vi "Ballard - 1553 - Main Page.vi"(8 "error in (no error)":errorcluster, 11 "Node Ptr":T2 format="%.0x") -> (0 "error out":errorcluster)   [LabVIEW 2017, in "Ballard 1553 System Explorer.lvlib"]
uses:
  Ballard 1553 System Explorer.lvlib
  <vilib>/NI Veristand/Custom Device API/Custom Device Item Ref.ctl
  Shared/Controls and Global/Initialization Method.ctl
  Shared/Controls and Global/Global.vi
  <vilib>/NI Veristand/Custom Device API/Get Item Property (U16).vi
  <vilib>/NI Veristand/Custom Device API/Get Item Property (I32).vi
  <vilib>/NI Veristand/Custom Device API/Get Item Property (Path).vi
  <vilib>/NI Veristand/Custom Device API/Get Item Property (String).vi
  <vilib>/NI Veristand/Custom Device API/Set Item Property (I32).vi
  <vilib>/NI Veristand/Custom Device API/Set Item Property (U16).vi
  <vilib>/NI VeriStand/Custom Device API/Custom Device API.lvlib
  Shared/Ballard 1553 Shared.lvlib
panel:
  in  "PXI Slot Number":i32=1 min=1 max=18 step=1
  in  "Initialization Method":T1
  out "Parameters Configuration Warning text":string="WARNING: The Parameters Configuration File has changed since import. If you attempt to run this system definition an error may occur. Consider refreshing the database import."
  out "Parameters Configuration File":path
  in  "Core Number":i32
  in  "Card Number":i32 min=0 max=18 step=1
  out "Version":string
  out "HW Configuration Warning text":string="WARNING: The database has changed since import. If you attempt to run this system definition an error may occur. Consider refreshing the database import."
  out "Warn Icon":bool
  out "Hardware Configuration File":path
  in  "Header":cluster{"Section Name":string}={"Section Name"="Ballard - MIL-STD-1553 - Custom Device"}
  in  "Description":string
  in  "Name":string
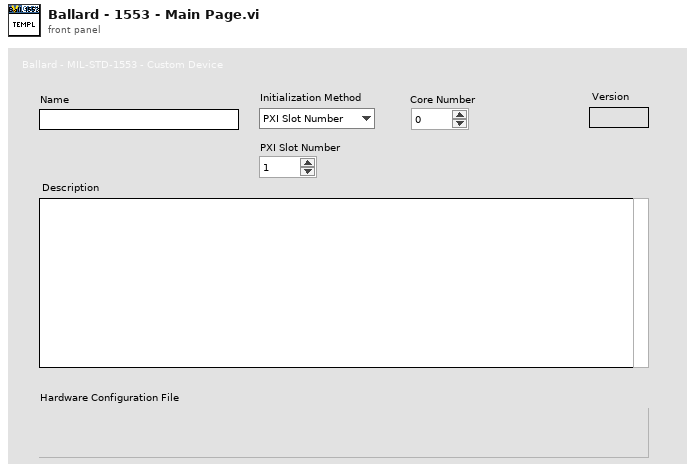
[diagram p1: front panel]
types:
  T1 = typedef "Ballard 1553 Shared.lvlib/Initialization Method.ctl" = enum16{"PXI Slot Number", "Card Number"}
  T2 = typedef "Custom Device API.lvlib/Custom Device Item Ref.ctl" = u64
  T3 = typedef "Custom Device API.lvlib/Custom Device Item Info.ctl" = cluster{"Name":string, "Is Channel":bool, "GUID":string, "Is Waveform":bool}
  T4 = typedef "Custom Device API.lvlib/Custom Device Commands.ctl" = enum16{"Default", "Item renamed", "Shutdown", "Dynamic button pressed"}
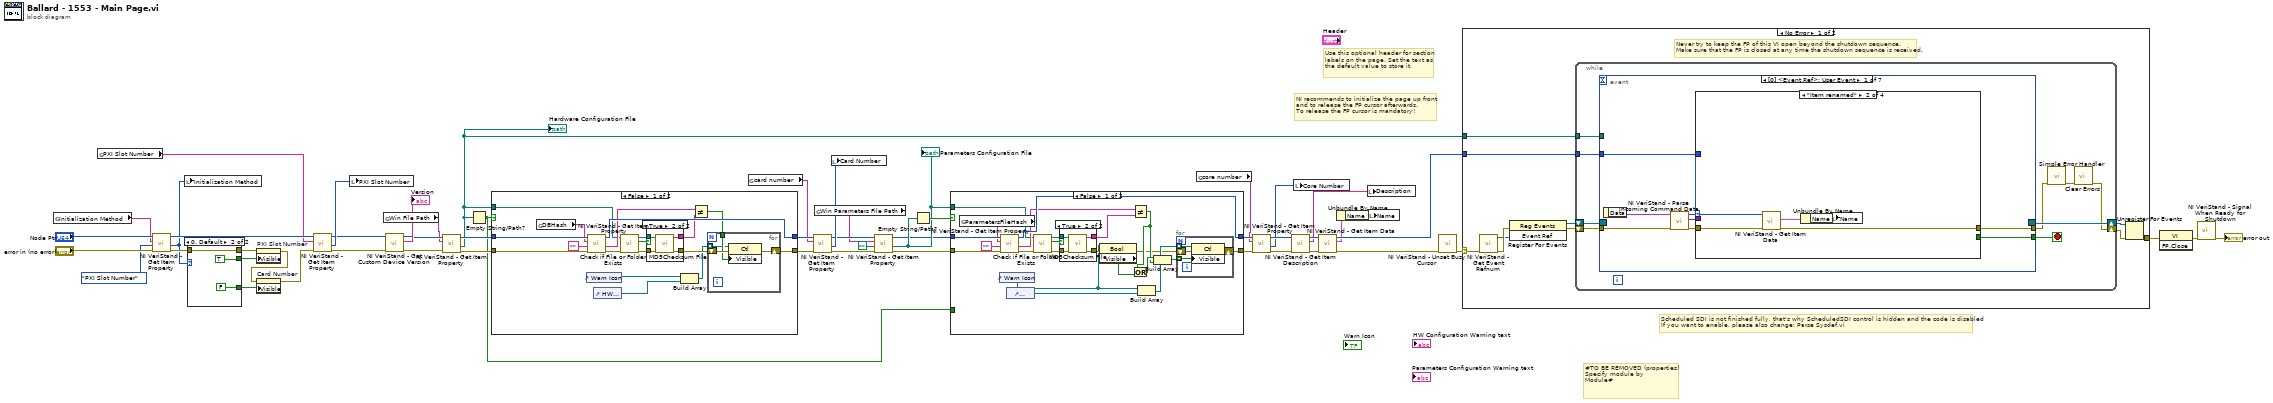
[diagram p0: block diagram]
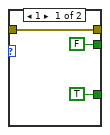
[diagram p2: hidden frame]
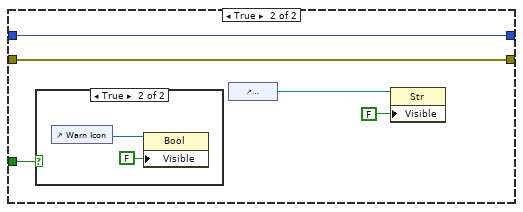
[diagram p4: hidden frame]
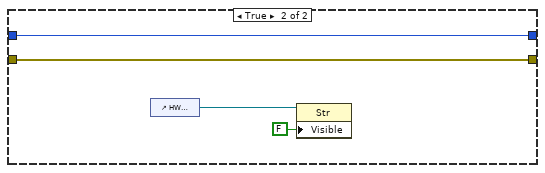
[diagram p7: hidden frame]
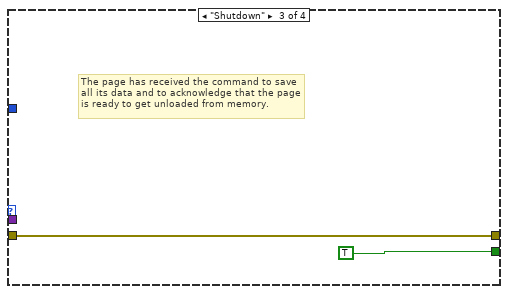
[diagram p9: hidden frame]
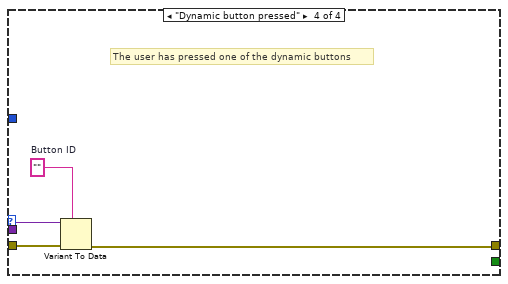
[diagram p10: hidden frame]
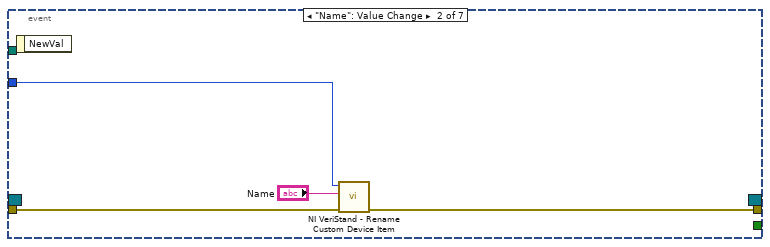
[diagram p11: hidden frame]
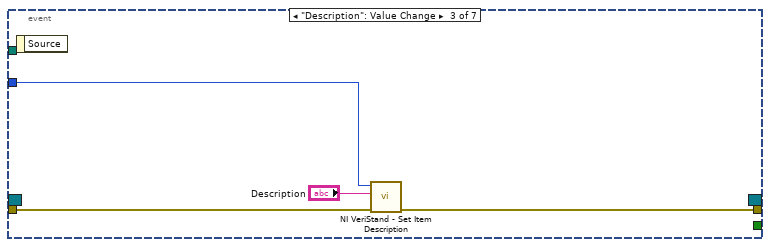
[diagram p12: hidden frame]
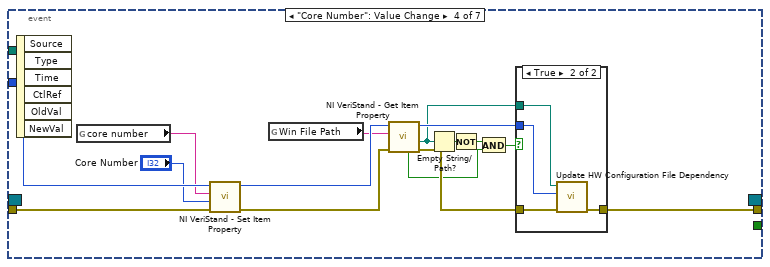
[diagram p13: hidden frame]
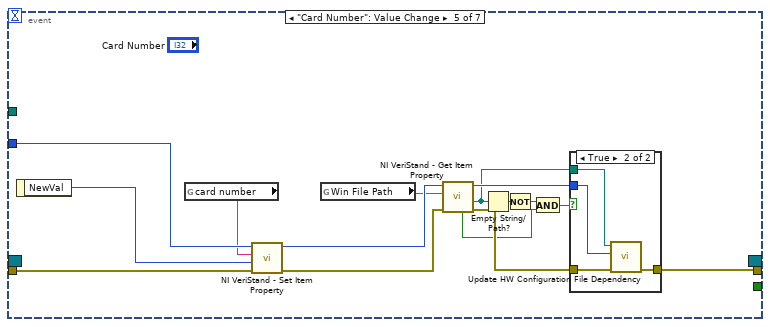
[diagram p15: hidden frame]
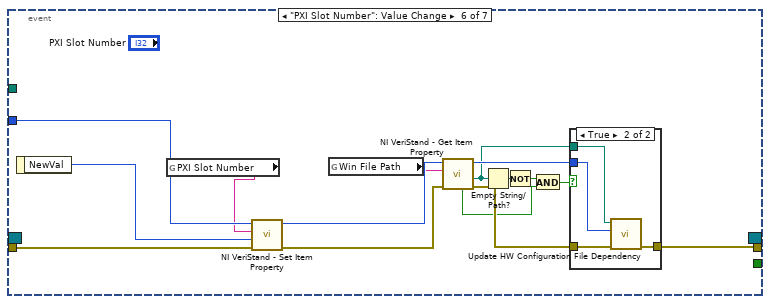
[diagram p17: hidden frame]
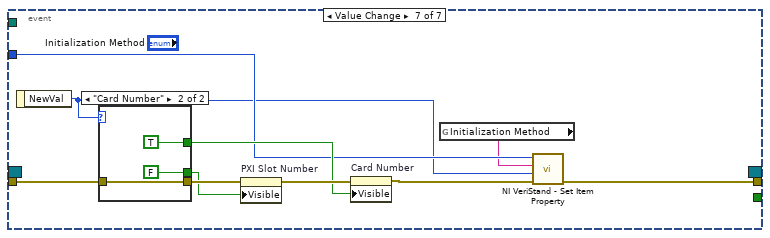
[diagram p19: hidden frame]
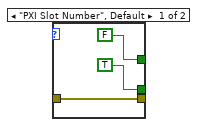
[diagram p20: hidden frame]
diagram:
  # "#TO BE REMOVED (properties)\nSpecify module by\nModule#"
  # "Scheduled SDI is not finished fully, that's why ScheduledSDI control is hidden and the code is disabled\nIf you want to enable, please also change: Parse Sysdef.vi"
  # "Use this optional header for section labels on the page. Set the text as the default value to store it."
  # "NI recommends to initialize the page up front\nand to release the FP cursor afterwards.\nTo release the FP cursor is mandatory!"
  n1 = global read "Global.vi" "Initialization Method"() -> (w5:string)
  n2 = global read "Global.vi" "PXI Slot Number"() -> (w6:string)
  n3 = call-poly <vilib>:"NI VeriStand - Get Item Property.vi"("error in (no error)"="error in (no error)", "Default Value"=Initialization_Method."PXI Slot Number" ("Initialization Method"), "Property Name"=w5, "Item Ref in"="Node Ptr") -> ("error out"=w13:errorcluster, "Value"=w12:u16, "Item Ref out"=w20:T2)  [unwired: 4 in, 1 out]
  n4 = local write "Initialization Method"(w12) -> ()
  n5 = case shown="0, Default" w12 {
    tunnel: w13 -> [w56 w59]
    tunnel: [FALSE TRUE] -> w11
    tunnel: [w56 w59] -> w10
    tunnel: [TRUE FALSE] -> w7
    frame 1 {
    }
    frame 0, Default {
    }
  }
  n6 = property on="PXI Slot Number" class="DigNum (strict)"(error in=w10, "Visible"=w11) -> (error out=w9:errorcluster)  [unwired: 1 in, 1 out]
  n7 = property on="Card Number" class="DigNum (strict)"(error in=w9, "Visible"=w7) -> (error out=w8:errorcluster)  [unwired: 1 in, 1 out]
  n8 = call-poly <vilib>:"NI VeriStand - Get Item Property.vi"("error in (no error)"=w8, "Property Name"=w6, "Item Ref in"=w20) -> ("error out"=w14:errorcluster, "Value"=w16:i32, "Item Ref out"=w15:T2)  [unwired: 5 in, 1 out]
  n9 = local write "PXI Slot Number"(w16) -> ()
  n10 = global read "Global.vi" "Win File Path"() -> (w4:string)
  n11 = call <vilib>:"NI VeriStand - Get Custom Device Version.vi"("error in (no error)"=w14, "Device Ref in"=w15) -> ("error out"=w35:errorcluster, "Value"=→"Version":string, "Device Ref out"=w36:T2)  [unwired: 7 in]
  n12 = call-poly <vilib>:"NI VeriStand - Get Item Property.vi"("error in (no error)"=w35, "Property Name"=w4, "Item Ref in"=w36) -> ("error out"=w42:errorcluster, "Value"=w38:path, "Item Ref out"=w39:T2)  [unwired: 5 in, 1 out]
  "Hardware Configuration File" <- w38
  n13 = Empty String/Path?(string/path=w38) -> (empty?=w21:bool)
  n14 = case shown="False" w21 {
    tunnel: w42 -> [w75 w90]
    tunnel: [w66 w90] -> w41
    tunnel: [w74 w89] -> w40
    tunnel: w39 -> [w76 w89]
    tunnel: w38 -> [w62 _]
    frame False {
      n15 = global read "Global.vi" "DBHash"() -> (w60:string)
      n16 = control-ref of="Warn Icon"() -> (w68:refnum<vi>)
      n17 = call-poly <vilib>:"NI VeriStand - Get Item Property.vi"("error in (no error)"=w75, "Default Value"="", "Property Name"=w60, "Item Ref in"=w76) -> ("error out"=w63:errorcluster, "Value"=w72:string, "Item Ref out"=w74:T2)  [unwired: 4 in, 1 out]
      n18 = control-ref of="HW Configuration Warning text"() -> (w69:refnum<vi>)
      n19 = call <vilib>:"Check if File or Folder Exists.vi"("error in (no error)"=w63, "path"=w62) -> ("error out"=w65:errorcluster, "file or folder exists?"=w61:bool, "dup path"=w64:path)  [unwired: 7 in]
      n20 = case shown="True" w61 {
        tunnel: [_ w82] -> w73
        tunnel: [w78 w81] -> w71
        tunnel: w65 -> [w78 w80]
        tunnel: w64 -> [_ w79]
        frame False {
        }
        frame True {
          n21 = call <vilib>:"MD5Checksum File.vi"("error in (no error)"=w80, "Path"=w79) -> ("error out"=w81:errorcluster, "MD5 message-digest"=w82:string)  [unwired: 8 in]
        }
      }
      n22 = Build Array(w68, w69) -> (w67:refnum<vi>[])
      n23 = Not Equal?(x=w72, y=w73) -> (x != y?=w70:bool)
      n24 = for {
        shift-right: [w85] -> w66
        shift-left: w71 -> [w86]
        tunnel: w70 -> [w84]
        tunnel: w67 -> [w83] mode=indexing
        n25 = property class="Ctl"(reference=w83, error in=w86, "Visible"=w84) -> (error out=w85:errorcluster)  [unwired: 1 out]
      }
    }
    frame True {
      n26 = control-ref of="HW Configuration Warning text"() -> (w88:refnum<vi>)
      n27 = property class="Str"(reference=w88, "Visible"=FALSE) -> ()  [unwired: 1 in, 2 out]
    }
  }
  n28 = global read "Global.vi" "card number"() -> (w3:string)
  n29 = call-poly <vilib>:"NI VeriStand - Get Item Property.vi"("error in (no error)"=w41, "Property Name"=w3, "Item Ref in"=w40) -> ("error out"=w29:errorcluster, "Value"=w31:i32, "Item Ref out"=w30:T2)  [unwired: 5 in, 1 out]
  n30 = global read "Global.vi" "Win Parameters File Path"() -> (w2:string)
  n31 = local write "Card Number"(w31) -> ()
  n32 = call-poly <vilib>:"NI VeriStand - Get Item Property.vi"("error in (no error)"=w29, "Default Value"=path "", "Property Name"=w2, "Item Ref in"=w30) -> ("error out"=w24:errorcluster, "Value"=w27:path, "Item Ref out"=w26:T2)  [unwired: 4 in, 1 out]
  "Parameters Configuration File" <- w27
  n33 = Empty String/Path?(string/path=w27) -> (empty?=w28:bool)
  n34 = case shown="False" w28 {
    tunnel: [w107 w125] -> w23
    tunnel: [w110 w126] -> w25
    tunnel: w26 -> [w111 w126]
    tunnel: w27 -> [w103 _]
    tunnel: w24 -> [w92 w125]
    tunnel: w21 -> [_ w122]
    frame False {
      n35 = global read "Global.vi" "ParametersFileHash"() -> (w91:string)
      n36 = control-ref of="Warn Icon"() -> (w93:refnum<vi>)
      n37 = call-poly <vilib>:"NI VeriStand - Get Item Property.vi"("error in (no error)"=w92, "Default Value"="", "Property Name"=w91, "Item Ref in"=w111) -> ("error out"=w104:errorcluster, "Value"=w108:string, "Item Ref out"=w110:T2)  [unwired: 4 in, 1 out]
      n38 = control-ref of="Parameters Configuration Warning text"() -> (w101:refnum<vi>)
      n39 = call <vilib>:"Check if File or Folder Exists.vi"("error in (no error)"=w104, "path"=w103) -> ("error out"=w106:errorcluster, "file or folder exists?"=w102:bool, "dup path"=w105:path)  [unwired: 7 in]
      n40 = case shown="True" w102 {
        tunnel: [_ w121] -> w109
        tunnel: [w117 w120] -> w98
        tunnel: w106 -> [w117 w119]
        tunnel: w105 -> [_ w118]
        frame False {
        }
        frame True {
          n41 = call <vilib>:"MD5Checksum File.vi"("error in (no error)"=w119, "Path"=w118) -> ("error out"=w120:errorcluster, "MD5 message-digest"=w121:string)  [unwired: 8 in]
        }
      }
      n42 = property class="Bool"(reference=w93, error in=w98) -> (error out=w94:errorcluster, "Visible"=w96:bool)  [unwired: 1 out]
      n43 = Not Equal?(x=w108, y=w109) -> (x != y?=w95:bool)
      n44 = Or(x=w95, y=w96) -> (x .or. y?=w97:bool)
      n45 = Build Array(w93, w101) -> (w100:refnum<vi>[])
      n46 = Build Array(w97, w95) -> (w99:bool[])
      n47 = for {
        tunnel: w99 -> [w114] mode=indexing
        shift-right: [w115] -> w107
        shift-left: w94 -> [w116]
        tunnel: w100 -> [w113] mode=indexing
        n48 = property class="Ctl"(reference=w113, error in=w116, "Visible"=w114) -> (error out=w115:errorcluster)  [unwired: 1 out]
      }
    }
    frame True {
      n49 = case shown="True" w122 {
        frame False {
        }
        frame True {
          n50 = control-ref of="Warn Icon"() -> (w128:refnum<vi>)
          n51 = property class="Bool"(reference=w128, "Visible"=FALSE) -> ()  [unwired: 1 in, 2 out]
        }
      }
      n52 = control-ref of="Parameters Configuration Warning text"() -> (w124:refnum<vi>)
      n53 = property class="Str"(reference=w124, "Visible"=FALSE) -> ()  [unwired: 1 in, 2 out]
    }
  }
  n54 = global read "Global.vi" "core number"() -> (w1:string)
  n55 = call-poly <vilib>:"NI VeriStand - Get Item Property.vi"("error in (no error)"=w23, "Property Name"=w1, "Item Ref in"=w25) -> ("error out"=w34:errorcluster, "Value"=w32:i32, "Item Ref out"=w33:T2)  [unwired: 5 in, 1 out]
  n56 = call <vilib>:"NI VeriStand - Get Item Description.vi"("error in (no error)"=w34, "Item Ref in"=w33) -> ("error out"=w45:errorcluster, "Description"=w46:string, "Item Ref out"=w47:T2)  [unwired: 7 out]
  n57 = local write "Core Number"(w32) -> ()
  n58 = call <vilib>:"NI VeriStand - Get Item Data.vi"("error in (no error)"=w45, "Item Ref in"=w47) -> ("error out"=w50:errorcluster, "Item Info"=w44:T3, "Item Ref out"=w48:T2)  [unwired: 7 out]
  n59 = Unbundle By Name(w44) -> ("Name"=w43:string)
  n60 = local write "Description"(w46) -> ()
  n61 = local write "Name"(w43) -> ()
  n62 = call <vilib>:"NI VeriStand - Unset Busy Cursor.vi"("error in (no error)"=w50) -> ("error out"=w49:errorcluster)  [unwired: 10 out]
  n63 = case shown="No Error" w49 {
    selector: w49 -> [w130 w254]
    tunnel: [w135 w252] -> w53
    tunnel: w48 -> [w131 _]
    tunnel: w38 -> [w129 _]
    frame No Error {
      # "Never try to keep the FP of this VI open beyond the shutdown sequence.\nMake sure that the FP is closed at any time the shutdown sequence is received."
      n64 = call <vilib>:"NI VeriStand - Get Event Refnum.vi"("error in (no error)"=w130) -> ("error out"=w138:errorcluster, "Event Ref"=w134:refnum<user-event>)  [unwired: 9 out]
      n65 = register-events(error in=w138, w134) -> (reference out=w132:refnum<event-registration>, error out=w133:errorcluster)  [unwired: 1 in]
      n66 = while {
        tunnel: w131 -> [w143]
        shift-right: [w140] -> w136
        shift-left: w133 -> [w146]
        shift-right: [w147] -> w137
        shift-left: w132 -> [w145]
        tunnel: w129 -> [w139]
        stop <- w144 stop-if-true
        n67 = event shown="[0] <Event Ref>: User Event" {
          selector: w145 -> [_ _ _ _ _ _ _]
          dyn-events: [_ _ _ _ _ _ _] -> w147
          timeout: _ -> [_ _ _ _ _ _ _]
          tunnel: w146 -> [w155 w171 w174 w190 w210 w230 w245]
          tunnel: [w151 _ _ _ _ _ _] -> w144
          tunnel: [w150 w170 w173 w179 w203 w223 w237] -> w142
          tunnel: w143 -> [w149 w169 w175 w189 w209 w229 w240]
          tunnel: w139 -> [_ _ _ _ _ _ _]
          event User Event {
            n68 = event-data() -> ("Data"=w154:string)  [unwired: 1 out]
            n69 = call <vilib>:"NI VeriStand - Parse Incoming Command Data.vi"("error in (no error)"=w155, "Incoming data"=w154) -> ("error out"=w153:errorcluster, "Outgoing data"=w148:variant, "Action"=w152:T4)  [unwired: 7 out]
            n70 = case shown="\"Item renamed\"" w152 {
              tunnel: w153 -> [w156 w161 w162 w167]
              tunnel: [_ _ TRUE _] -> w151
              tunnel: [w156 w158 w162 w164] -> w150
              tunnel: w149 -> [_ w160 _ _]
              tunnel: w148 -> [_ _ _ w166]
              frame "Default", Default {
              }
              frame "Item renamed" {
                n71 = call <vilib>:"NI VeriStand - Get Item Data.vi"("error in (no error)"=w161, "Item Ref in"=w160) -> ("error out"=w158:errorcluster, "Item Info"=w159:T3)  [unwired: 8 out]
                n72 = Unbundle By Name(w159) -> ("Name"=w157:string)
                n73 = local write "Name"(w157) -> ()
              }
              frame "Shutdown" {
                # "The page has received the command to save all its data and to acknowledge that the page is ready to get unloaded from memory."
              }
              frame "Dynamic button pressed" {
                w165 = ""  # Button ID
                # "The user has pressed one of the dynamic buttons"
                n74 = Variant To Data(error in=w167, type=w165, Variant=w166) -> (error out=w164:errorcluster)  [unwired: 1 out]
              }
            }
          }
          event "Name": Value Change {
            n75 = event-data() -> ()  [unwired: 2 out]
            n76 = call <vilib>:"NI VeriStand - Rename Custom Device Item.vi"("error in (no error)"=w171, "New Name"="Name", "Item Ref in"=w169) -> ("error out"=w170:errorcluster)  [unwired: 1 in, 7 out]
          }
          event "Description": Value Change {
            n77 = event-data() -> ()  [unwired: 2 out]
            n78 = call <vilib>:"NI VeriStand - Set Item Description.vi"("error in (no error)"=w174, "Description"="Description", "Item Ref in"=w175) -> ("error out"=w173:errorcluster)  [unwired: 8 out]
          }
          event "Core Number": Value Change {
            n79 = event-data() -> ()  [unwired: 7 out]
            n80 = global read "Global.vi" "core number"() -> (w177:string)
            n81 = call-poly <vilib>:"NI VeriStand - Set Item Property.vi"("error in (no error)"=w190, "Value"="Core Number", "Property Name"=w177, "Item Ref in"=w189) -> ("error out"=w181:errorcluster, "Item Ref out"=w180:T2)  [unwired: 5 in, 1 out]
            n82 = global read "Global.vi" "Win File Path"() -> (w176:string)
            n83 = call-poly <vilib>:"NI VeriStand - Get Item Property.vi"("error in (no error)"=w181, "Property Name"=w176, "Item Ref in"=w180) -> ("error out"=w187:errorcluster, "Value"=w178:path, "Item Ref out"=w186:T2, "Found?"=w184:bool)  [unwired: 5 in]
            n84 = Empty String/Path?(string/path=w178) -> (empty?=w185:bool)
            n85 = Not(x=w185) -> (.not. x?=w182:bool)
            n86 = And(x=w182, y=w184) -> (x .and. y?=w183:bool)
            n87 = case shown="True" w183 {
              tunnel: [w191 w195] -> w179
              tunnel: w187 -> [w191 w194]
              tunnel: w186 -> [_ w193]
              tunnel: w178 -> [_ w192]
              frame False {
              }
              frame True {
                n88 = call "Update HW Configuration File Dependency.vi"("error in (no error)"=w194, "Node Ptr dup"=w193, "selected path in"=w192) -> ("error out"=w195:errorcluster)  [unwired: 8 in]
              }
            }
          }
          event "Card Number": Value Change {
            n89 = event-data() -> ("NewVal"=w208:i32)  [unwired: 1 out]
            n90 = global read "Global.vi" "card number"() -> (w197:string)
            n91 = call-poly <vilib>:"NI VeriStand - Set Item Property.vi"("error in (no error)"=w210, "Value"=w208, "Property Name"=w197, "Item Ref in"=w209) -> ("error out"=w205:errorcluster, "Item Ref out"=w204:T2)  [unwired: 5 in, 1 out]
            n92 = global read "Global.vi" "Win File Path"() -> (w196:string)
            n93 = call-poly <vilib>:"NI VeriStand - Get Item Property.vi"("error in (no error)"=w205, "Property Name"=w196, "Item Ref in"=w204) -> ("error out"=w207:errorcluster, "Value"=w198:path, "Item Ref out"=w206:T2, "Found?"=w201:bool)  [unwired: 5 in]
            n94 = Empty String/Path?(string/path=w198) -> (empty?=w202:bool)
            n95 = Not(x=w202) -> (.not. x?=w199:bool)
            n96 = And(x=w199, y=w201) -> (x .and. y?=w200:bool)
            n97 = case shown="True" w200 {
              tunnel: [w211 w215] -> w203
              tunnel: w207 -> [w211 w214]
              tunnel: w206 -> [_ w213]
              tunnel: w198 -> [_ w212]
              frame False {
              }
              frame True {
                n98 = call "Update HW Configuration File Dependency.vi"("error in (no error)"=w214, "Node Ptr dup"=w213, "selected path in"=w212) -> ("error out"=w215:errorcluster)  [unwired: 8 in]
              }
            }
          }
          event "PXI Slot Number": Value Change {
            n99 = event-data() -> ("NewVal"=w228:i32)  [unwired: 1 out]
            n100 = global read "Global.vi" "PXI Slot Number"() -> (w216:string)
            n101 = call-poly <vilib>:"NI VeriStand - Set Item Property.vi"("error in (no error)"=w230, "Value"=w228, "Property Name"=w216, "Item Ref in"=w229) -> ("error out"=w225:errorcluster, "Item Ref out"=w224:T2)  [unwired: 5 in, 1 out]
            n102 = global read "Global.vi" "Win File Path"() -> (w217:string)
            n103 = call-poly <vilib>:"NI VeriStand - Get Item Property.vi"("error in (no error)"=w225, "Property Name"=w217, "Item Ref in"=w224) -> ("error out"=w227:errorcluster, "Value"=w218:path, "Item Ref out"=w226:T2, "Found?"=w221:bool)  [unwired: 5 in]
            n104 = Empty String/Path?(string/path=w218) -> (empty?=w222:bool)
            n105 = Not(x=w222) -> (.not. x?=w219:bool)
            n106 = And(x=w219, y=w221) -> (x .and. y?=w220:bool)
            n107 = case shown="True" w220 {
              tunnel: [w231 w235] -> w223
              tunnel: w227 -> [w231 w234]
              tunnel: w226 -> [_ w233]
              tunnel: w218 -> [_ w232]
              frame False {
              }
              frame True {
                n108 = call "Update HW Configuration File Dependency.vi"("error in (no error)"=w234, "Node Ptr dup"=w233, "selected path in"=w232) -> ("error out"=w235:errorcluster)  [unwired: 8 in]
              }
            }
          }
          event Value Change {
            n109 = event-data() -> ("NewVal"=w239:T1)  [unwired: 1 out]
            n110 = case shown="\"Card Number\"" w239 {
              tunnel: w245 -> [w248 w251]
              tunnel: [w248 w251] -> w244
              tunnel: [FALSE TRUE] -> w242
              tunnel: [TRUE FALSE] -> w241
              frame "PXI Slot Number", Default {
              }
              frame "Card Number" {
              }
            }
            n111 = property on="PXI Slot Number" class="DigNum (strict)"(error in=w244, "Visible"=w241) -> (error out=w243:errorcluster)  [unwired: 1 in, 1 out]
            n112 = property on="Card Number" class="DigNum (strict)"(error in=w243, "Visible"=w242) -> (error out=w238:errorcluster)  [unwired: 1 in, 1 out]
            n113 = global read "Global.vi" "Initialization Method"() -> (w236:string)
            n114 = call-poly <vilib>:"NI VeriStand - Set Item Property.vi"("error in (no error)"=w238, "Value"=w239, "Property Name"=w236, "Item Ref in"=w240) -> ("error out"=w237:errorcluster)  [unwired: 5 in, 2 out]
          }
        }
        n115 = call <vilib>:"Simple Error Handler.vi"("error in (no error)"=w142) -> ("error out"=w141:errorcluster)  [unwired: 1 in, 7 out]
        n116 = call <vilib>:"Clear Errors.vi"("error in (no error)"=w141) -> ("error out"=w140:errorcluster)  [unwired: 1 in, 5 out]
      }
      n117 = Unregister For Events(event registration refnum=w137, error in=w136) -> (error out=w135:errorcluster)
    }
    frame Error {
      n118 = call <vilib>:"Simple Error Handler.vi"("error in (no error)"=w254) -> ("error out"=w253:errorcluster)  [unwired: 1 in, 7 out]
      n119 = call <vilib>:"Clear Errors.vi"("error in (no error)"=w253) -> ("error out"=w252:errorcluster)  [unwired: 1 in, 5 out]
    }
  }
  n120 = invoke class="VI" method="FP.Close"(error in=w53) -> (error out=w52:errorcluster)  [unwired: 2 in, 2 out]
  n121 = call <vilib>:"NI VeriStand - Signal When Ready for Shutdown.vi"("error in (no error)"=w52) -> ("error out"=→"error out":errorcluster)  [unwired: 10 out]
